vi "Throw -8715 error.vi"(8 "error in (no error)":errorcluster, 10 "Custom device name":string, 11 "Error":bool) -> (0 "error out":errorcluster)   [LabVIEW 2019, in "Engine Simulation Toolkit System Explorer.lvlib"]
uses:
  Engine Simulation Toolkit System Explorer.lvlib
  <vilib>/Utility/error.llb/Error Cluster From Error Code.vi
  <vilib>/ErrorRing/Error Ring.xnode
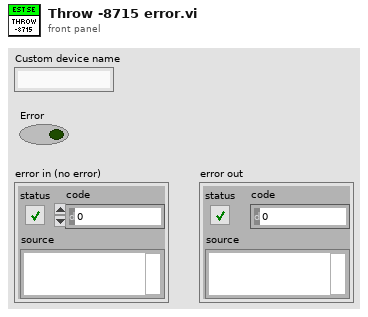
[diagram p1: front panel]
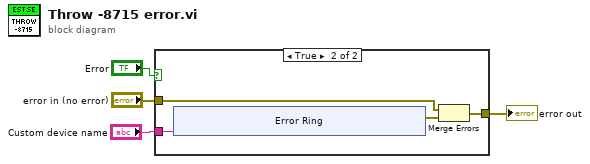
[diagram p0: block diagram]
diagram:
  n1 = case shown="True" "Error" {
    tunnel: "error in (no error)" -> [w5 w9]
    tunnel: "Custom device name" -> [_ w7]
    tunnel: [w5 w6] -> w4
    frame False {
    }
    frame True {
      n2 = xnode "Error Ring"("parameter 0"=w7) -> ("error out"=w8:errorcluster)
      n3 = Merge Errors(w9, w8) -> (w6:errorcluster)
    }
  }
  "error out" <- w4
